vi "Perimeter.vi"(8 "error in (no error)":errorcluster, 11 "Square in":refnum<class "Square.lvclass">) -> (0 "error out":errorcluster, 2 "perimeter":dbl, 3 "Square out":refnum<class "Square.lvclass">)   [LabVIEW 2015, in "Square.lvclass"]
uses:
  Square.lvclass
  Square.lvclass/Square.ctl
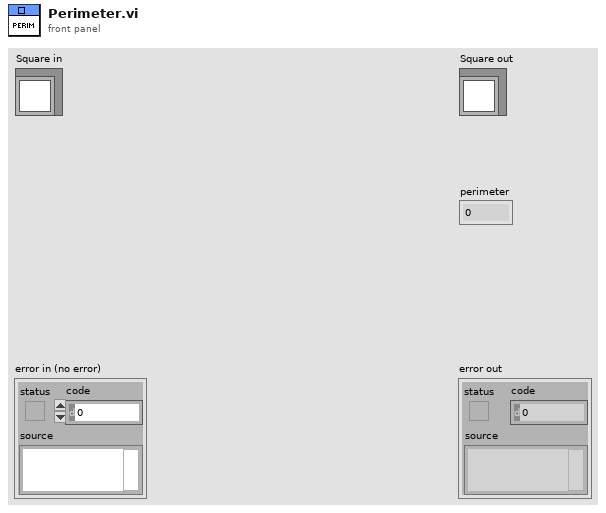
[diagram p1: front panel]
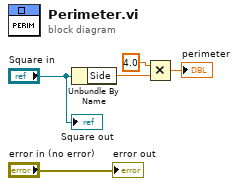
[diagram p0: block diagram]
diagram:
  n1 = Unbundle By Name("Square in") -> ("Side"=w5:dbl)
  n2 = Multiply(x=4.0, y=w5) -> (x*y=→"perimeter":dbl)
  "error out" <- "error in (no error)"
  "Square out" <- "Square in"
